vi "Method.vi"(4 "Input B":refnum<class "Abs_Numeric.lvclass">, 5 "Input A":T1) -> (1 "Result":T1)   [LabVIEW 2021, in "Add_CPLX_DBL.lvclass"]
uses:
  Add_CPLX_DBL.lvclass
  Abs_Type.ctl
  Abs_Types/Complex Double Float/Complex Double Float.lvclass
  Abs_Types/Numeric/Abs_Numeric.lvclass
  C:/Users/Tim/Documents/LabVIEW/2021/Data Classes/Source/Functions/Support/Two Terminal/Cmplx DBL/AbsFunc_Two Term_Complex DBL.lvclass
  C:/Users/Tim/Documents/LabVIEW/2021/Data Classes/Source/Abs_Types/Complex Double Float/Complex Double Float.lvclass
  Support/Two Terminal/Cmplx DBL/AbsFunc_Two Term_Complex DBL.lvclass/AbsFunc_Two Term_Complex DBL.ctl
  Support/Two Terminal/Cmplx DBL/Properties/Write Numeric A.vi
  Support/Two Terminal/Cmplx DBL/Properties/Write Numeric B.vi
  Add_CPLX_DBL.lvclass/Add_CPLX_DBL.ctl
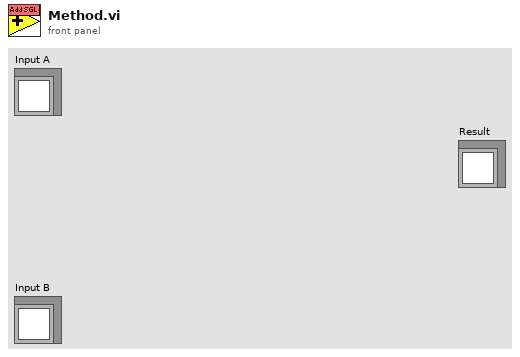
[diagram p1: front panel]
types:
  T1 = typedef "Add_CPLX_DBL.lvclass/Abs_Type.ctl" = refnum<class "Complex Double Float.lvclass">
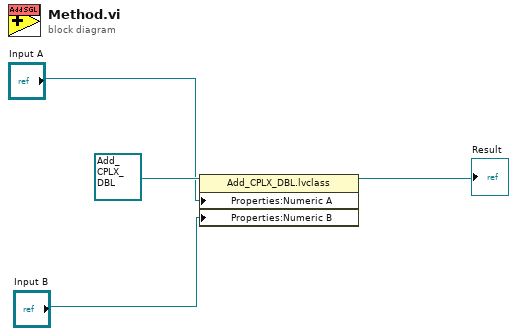
[diagram p0: block diagram]
diagram:
  n1 = property class="Add_CPLX_DBL.lvclass"(reference=refnum<class "Add_CPLX_DBL.lvclass"> refnum ("Functions.lvlib:Numeric.lvlib:Add_SGL.lvclass"), "Properties:Numeric A"="Input A", "Properties:Numeric B"="Input B") -> (reference out=→"Result":refnum<class "Add_CPLX_DBL.lvclass">)  [unwired: 1 in, 1 out]
